vi "Lighthouse Monitoring & Control System 3.vi"() -> ()   [LabVIEW 2012]
uses:
  <vilib>/DAQmx/read.llb/DAQmx Read (Counter DBL 1Chan 1Samp).vi
  <vilib>/DAQmx/write.llb/DAQmx Write (Digital U8 1Chan 1Samp).vi
  <vilib>/DAQmx/write.llb/DAQmx Write (Digital 1D Bool NChan 1Samp 1Line).vi
  <vilib>/DAQmx/write.llb/DAQmx Write (Analog DBL 1Chan 1Samp).vi
  <vilib>/DAQmx/read.llb/DAQmx Read (Analog DBL 1Chan 1Samp).vi
  <vilib>/DAQmx/create/channels.llb/DAQmx Create Channel (CI-Count Edges).vi
  <vilib>/DAQmx/create/channels.llb/DAQmx Create Channel (DO-Digital Output).vi
  <vilib>/DAQmx/create/channels.llb/DAQmx Create Channel (AI-Voltage-Basic).vi
  <vilib>/DAQmx/create/channels.llb/DAQmx Create Channel (AO-Voltage-Basic).vi
  <vilib>/DAQmx/miscellaneous.llb/DAQmx Fill In Error Info.vi
panel:
  out "Array":bool[](array[boolean])
  out "Data to Write":u32=255 format="%x"
  out "Voltage":dbl
  in  "?":bool
  out "Slot Count":dbl
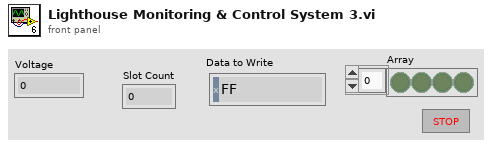
[diagram p1: front panel]
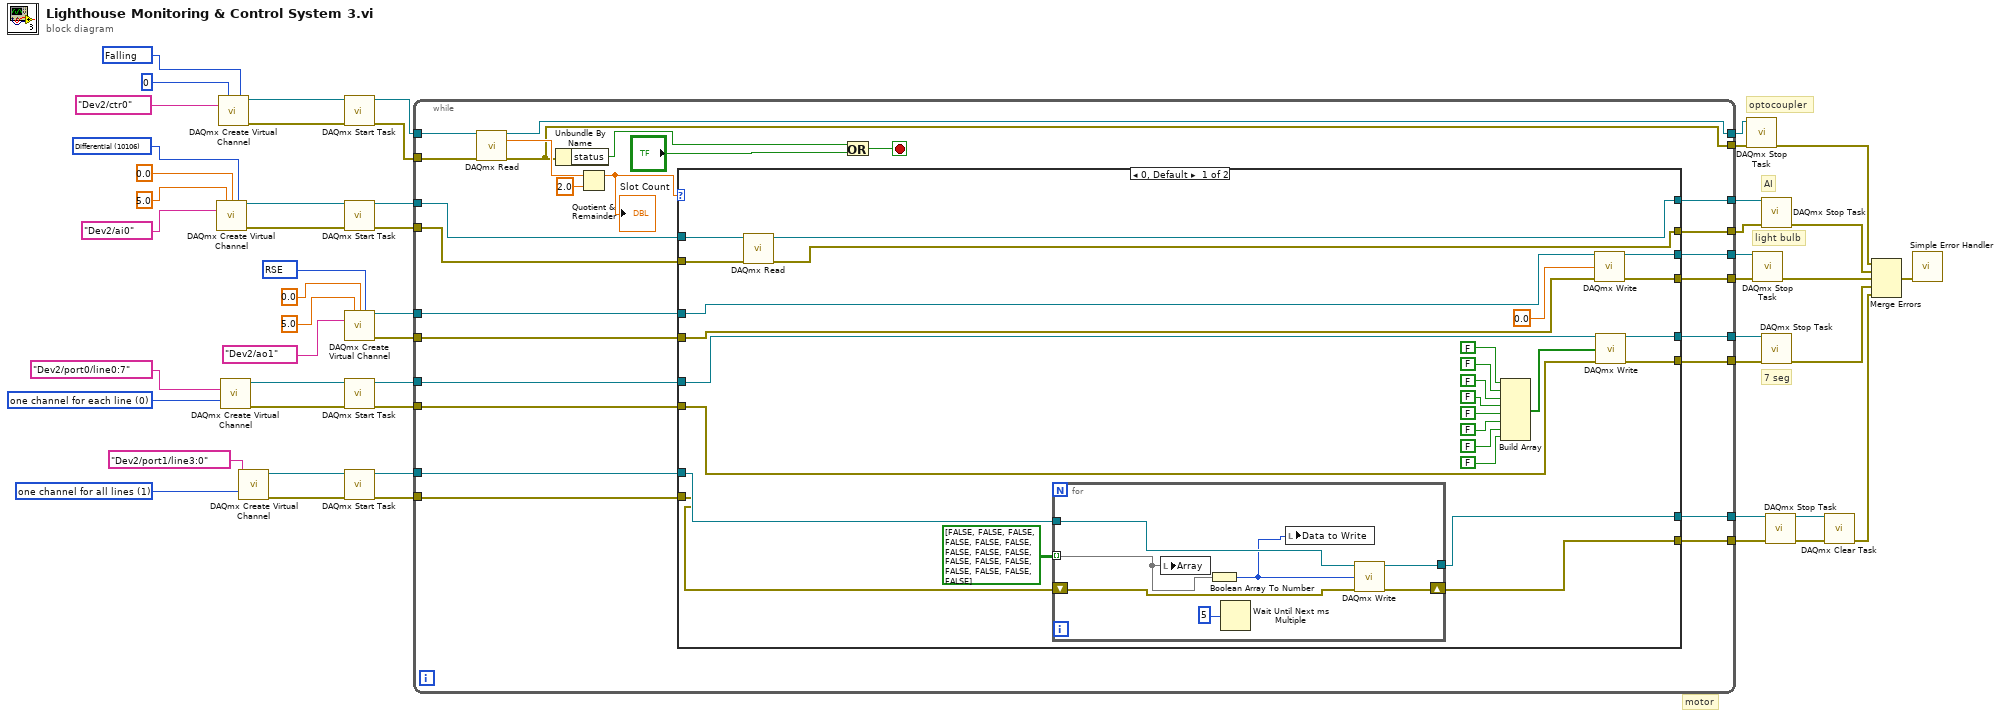
[diagram p0: block diagram]
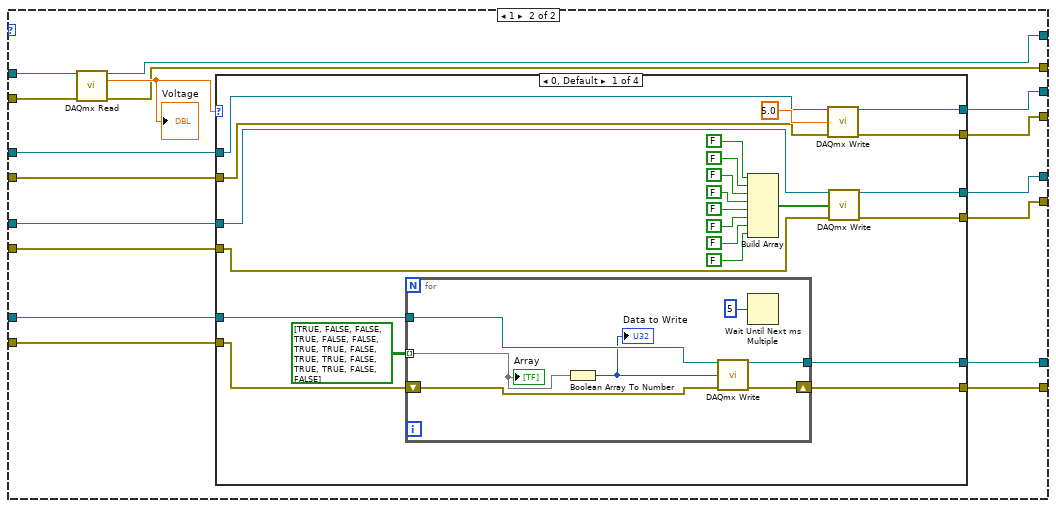
[diagram p2: hidden frame]
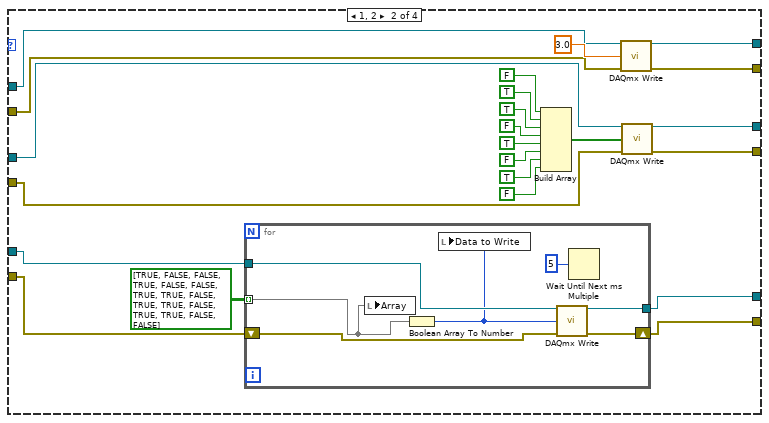
[diagram p3: hidden frame]
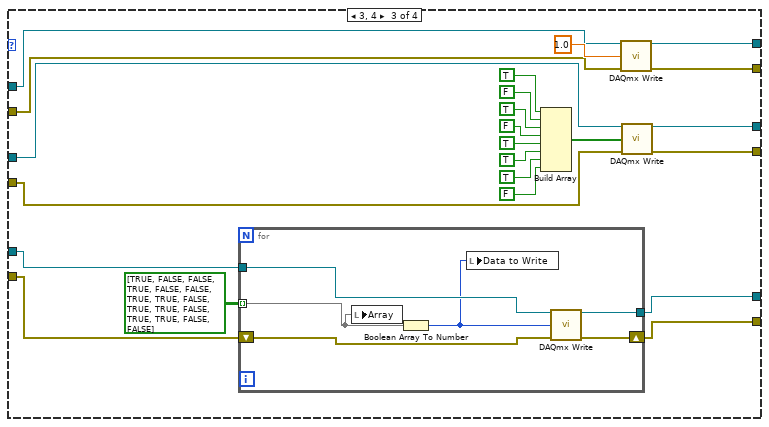
[diagram p4: hidden frame]
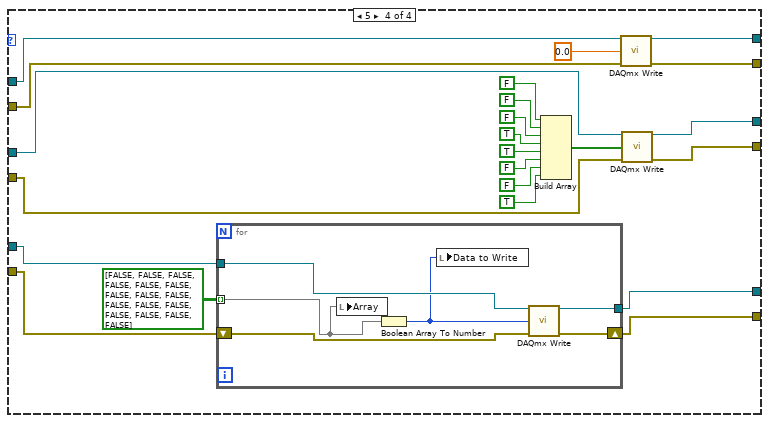
[diagram p5: hidden frame]
diagram:
  w11 = 1 items=["one channel for each line", "one channel for all lines"] ("line grouping")
  w38 = 0 items=["one channel for each line", "one channel for all lines"] ("line grouping")
  w41 = 10083 items=["Default"=-1, "RSE"=10083, "Differential"=10106, "Pseudodifferential"=12529] ("output terminal configuration")
  w44 = 10106 items=["default"=-1, "RSE"=10083, "NRSE"=10078, "Differential"=10106, "Pseudodifferential"=12529] ("input terminal configuration")
  w51 = 10171 items=["Rising"=10280, "Falling"=10171] ("edge")
  # "motor"
  # "7 seg"
  # "AI"
  # "light bulb"
  # "optocoupler"
  n1 = call-poly <vilib>:"DAQmx Create Virtual Channel.vi"("maximum value"=5.0, "minimum value"=0.0, "input terminal configuration"=w44, "physical channels"=tag "Dev2/ai0") -> ("task out"=w42:refnum<k21>, "error out"=w43:errorcluster)  [unwired: 10 in]
  n2 = call-poly <vilib>:"DAQmx Create Virtual Channel.vi"("initial count"=u32 0, "edge"=w51, "counter"=tag "Dev2/ctr0") -> ("task out"=w50:refnum<k21>, "error out"=w49:errorcluster)  [unwired: 11 in]
  n3 = call-poly <vilib>:"DAQmx Create Virtual Channel.vi"("lines"=tag "Dev2/port0/line0:7", "line grouping"=w38) -> ("task out"=w37:refnum<k21>, "error out"=w36:errorcluster)  [unwired: 12 in]
  n4 = call-poly <vilib>:"DAQmx Create Virtual Channel.vi"("lines"=tag "Dev2/port1/line3:0", "line grouping"=w11) -> ("task out"=w10:refnum<k21>, "error out"=w9:errorcluster)  [unwired: 12 in]
  n5 = call <vilib>:"DAQmx Start Task.vi"("task/channels in"=w50, "error in"=w49) -> ("task out"=w46:refnum<k21>, "error out"=w45:errorcluster)  [unwired: 12 in]
  n6 = call <vilib>:"DAQmx Start Task.vi"("task/channels in"=w42, "error in"=w43) -> ("task out"=w32:refnum<k21>, "error out"=w31:errorcluster)  [unwired: 12 in]
  n7 = call-poly <vilib>:"DAQmx Create Virtual Channel.vi"("maximum value"=5.0, "minimum value"=0.0, "output terminal configuration"=w41, "physical channels"=tag "Dev2/ao1") -> ("task out"=w30:refnum<k21>, "error out"=w29:errorcluster)  [unwired: 10 in]
  n8 = call <vilib>:"DAQmx Start Task.vi"("task/channels in"=w37, "error in"=w36) -> ("task out"=w28:refnum<k21>, "error out"=w27:errorcluster)  [unwired: 12 in]
  n9 = call <vilib>:"DAQmx Start Task.vi"("task/channels in"=w10, "error in"=w9) -> ("task out"=w8:refnum<k21>, "error out"=w7:errorcluster)  [unwired: 12 in]
  n10 = while {
    tunnel: w46 -> [w77]
    tunnel: w45 -> [w76]
    tunnel: [w64] -> w34
    tunnel: w32 -> [w70]
    tunnel: w31 -> [w69]
    tunnel: w30 -> [w68]
    tunnel: w29 -> [w67]
    tunnel: w28 -> [w66]
    tunnel: w27 -> [w65]
    tunnel: [w63] -> w22
    tunnel: [w62] -> w21
    tunnel: [w61] -> w20
    tunnel: [w60] -> w19
    tunnel: [w59] -> w18
    tunnel: [w58] -> w17
    tunnel: [w57] -> w16
    tunnel: w8 -> [w55]
    tunnel: w7 -> [w54]
    tunnel: [w52] -> w3
    tunnel: [w53] -> w2
    stop <- w73 stop-if-true
    n11 = call-poly <vilib>:"DAQmx Read.vi"("task/channels in"=w77, "error in"=w76) -> ("task out"=w64:refnum<k21>, "data"=w75:dbl, "error out"=w63:errorcluster)  [unwired: 11 in]
    n12 = Unbundle By Name(w63) -> ("status"=w72:bool)
    n13 = Quotient & Remainder(x=w75, y=2.0) -> (x-y*floor(x/y)=w56:dbl)  [unwired: 1 out]
    "Slot Count" <- w56
    n14 = case shown="0, Default" w56 {
      tunnel: w70 -> [w101 w127]
      tunnel: w69 -> [w100 w126]
      tunnel: w68 -> [w99 w125]
      tunnel: w67 -> [w98 w124]
      tunnel: w66 -> [w103 w123]
      tunnel: w65 -> [w102 w122]
      tunnel: [w95 w121] -> w58
      tunnel: [w96 w120] -> w62
      tunnel: [w97 w119] -> w61
      tunnel: [w92 w118] -> w60
      tunnel: [w93 w117] -> w59
      tunnel: [w94 w116] -> w57
      tunnel: w55 -> [w81 w115]
      tunnel: w54 -> [w80 w114]
      tunnel: [w78 w112] -> w53
      tunnel: [w79 w113] -> w52
      frame 0, Default {
        n15 = call-poly <vilib>:"DAQmx Read.vi"("task/channels in"=w101, "error in"=w100) -> ("task out"=w94:refnum<k21>, "error out"=w97:errorcluster)  [unwired: 11 in, 1 out]
        n16 = for {
          tunnel: w81 -> [w110]
          tunnel: [w109] -> w79
          shift-right: [w107] -> w78
          shift-left: w80 -> [w111]
          tunnel: bool[][] [[FALSE, FALSE, FALSE, FALSE], [FALSE, FALSE, FALSE, FALSE], [FALSE, FALSE, FALSE, FALSE], [FALSE, FALSE, FALSE, FALSE]] -> [w105] mode=indexing
          n17 = local write "Array"(w105) -> ()
          n18 = Boolean Array To Number(Boolean array=w105) -> (number=w106:u32)
          n19 = Wait Until Next ms Multiple(millisecond multiple=5) -> ()  [unwired: 1 out]
          n20 = local write "Data to Write"(w106) -> ()
          n21 = call-poly <vilib>:"DAQmx Write.vi"("task/channels in"=w110, "data"=w106, "error in"=w111) -> ("task out"=w109:refnum<k21>, "error out"=w107:errorcluster)  [unwired: 10 in, 1 out]
        }
        n22 = Build Array(FALSE, FALSE, FALSE, FALSE, FALSE, FALSE, FALSE, FALSE) -> (w83:bool[])
        n23 = call-poly <vilib>:"DAQmx Write.vi"("task/channels in"=w99, "data"=0.0, "error in"=w98) -> ("task out"=w95:refnum<k21>, "error out"=w96:errorcluster)  [unwired: 10 in, 1 out]
        n24 = call-poly <vilib>:"DAQmx Write.vi"("task/channels in"=w103, "data"=w83, "error in"=w102) -> ("task out"=w93:refnum<k21>, "error out"=w92:errorcluster)  [unwired: 10 in, 1 out]
      }
      frame 1 {
        n25 = call-poly <vilib>:"DAQmx Read.vi"("task/channels in"=w127, "error in"=w126) -> ("task out"=w116:refnum<k21>, "data"=w128:dbl, "error out"=w119:errorcluster)  [unwired: 11 in]
        "Voltage" <- w128
        n26 = case shown="0, Default" w128 {
          tunnel: w125 -> [w137 w171 w201 w230]
          tunnel: w124 -> [w136 w170 w200 w229]
          tunnel: [w141 w169 w199 w228] -> w121
          tunnel: [w140 w168 w198 w227] -> w120
          tunnel: [w139 w167 w197 w226] -> w117
          tunnel: [w138 w166 w196 w225] -> w118
          tunnel: w123 -> [w135 w165 w195 w224]
          tunnel: w122 -> [w134 w164 w194 w223]
          tunnel: w115 -> [w133 w162 w192 w221]
          tunnel: w114 -> [w132 w161 w191 w220]
          tunnel: [w131 w160 w190 w219] -> w113
          tunnel: [w130 w159 w189 w218] -> w112
          frame 0, Default {
            n27 = for {
              tunnel: w133 -> [w157]
              tunnel: [w156] -> w131
              shift-right: [w155] -> w130
              shift-left: w132 -> [w158]
              tunnel: bool[][] [[TRUE, FALSE, FALSE, TRUE], [FALSE, FALSE, TRUE, TRUE], [FALSE, TRUE, TRUE, FALSE], [TRUE, TRUE, FALSE, FALSE]] -> [w153] mode=indexing
              n28 = Boolean Array To Number(Boolean array=w153) -> (number=w154:u32)
              "Data to Write" <- w154
              n29 = call-poly <vilib>:"DAQmx Write.vi"("task/channels in"=w157, "data"=w154, "error in"=w158) -> ("task out"=w156:refnum<k21>, "error out"=w155:errorcluster)  [unwired: 10 in, 1 out]
              n30 = Wait Until Next ms Multiple(millisecond multiple=u32 5) -> ()  [unwired: 1 out]
              "Array" <- w153
            }
            n31 = Build Array(FALSE, FALSE, FALSE, FALSE, FALSE, FALSE, FALSE, FALSE) -> (w142:bool[])
            n32 = call-poly <vilib>:"DAQmx Write.vi"("task/channels in"=w137, "data"=5.0, "error in"=w136) -> ("task out"=w141:refnum<k21>, "error out"=w140:errorcluster)  [unwired: 10 in, 1 out]
            n33 = call-poly <vilib>:"DAQmx Write.vi"("task/channels in"=w135, "data"=w142, "error in"=w134) -> ("task out"=w139:refnum<k21>, "error out"=w138:errorcluster)  [unwired: 10 in, 1 out]
          }
          frame 1, 2 {
            n34 = for {
              tunnel: w162 -> [w183]
              tunnel: [w187] -> w160
              shift-right: [w186] -> w159
              shift-left: w161 -> [w188]
              tunnel: bool[][] [[TRUE, FALSE, FALSE, TRUE], [FALSE, FALSE, TRUE, TRUE], [FALSE, TRUE, TRUE, FALSE], [TRUE, TRUE, FALSE, FALSE]] -> [w184] mode=indexing
              n35 = local write "Array"(w184) -> ()
              n36 = Boolean Array To Number(Boolean array=w184) -> (number=w182:u32)
              n37 = local write "Data to Write"(w182) -> ()
              n38 = call-poly <vilib>:"DAQmx Write.vi"("task/channels in"=w183, "data"=w182, "error in"=w188) -> ("task out"=w187:refnum<k21>, "error out"=w186:errorcluster)  [unwired: 10 in, 1 out]
              n39 = Wait Until Next ms Multiple(millisecond multiple=u32 5) -> ()  [unwired: 1 out]
            }
            n40 = Build Array(FALSE, TRUE, TRUE, FALSE, TRUE, FALSE, TRUE, FALSE) -> (w172:bool[])
            n41 = call-poly <vilib>:"DAQmx Write.vi"("task/channels in"=w171, "data"=3.0, "error in"=w170) -> ("task out"=w169:refnum<k21>, "error out"=w168:errorcluster)  [unwired: 10 in, 1 out]
            n42 = call-poly <vilib>:"DAQmx Write.vi"("task/channels in"=w165, "data"=w172, "error in"=w164) -> ("task out"=w167:refnum<k21>, "error out"=w166:errorcluster)  [unwired: 10 in, 1 out]
          }
          frame 3, 4 {
            n43 = for {
              tunnel: w192 -> [w216]
              tunnel: [w215] -> w190
              shift-right: [w214] -> w189
              shift-left: w191 -> [w217]
              tunnel: bool[][] [[TRUE, FALSE, FALSE, TRUE], [FALSE, FALSE, TRUE, TRUE], [FALSE, TRUE, TRUE, FALSE], [TRUE, TRUE, FALSE, FALSE]] -> [w213] mode=indexing
              n44 = local write "Array"(w213) -> ()
              n45 = Boolean Array To Number(Boolean array=w213) -> (number=w212:u32)
              n46 = local write "Data to Write"(w212) -> ()
              n47 = call-poly <vilib>:"DAQmx Write.vi"("task/channels in"=w216, "data"=w212, "error in"=w217) -> ("task out"=w215:refnum<k21>, "error out"=w214:errorcluster)  [unwired: 10 in, 1 out]
            }
            n48 = Build Array(TRUE, FALSE, TRUE, FALSE, TRUE, TRUE, TRUE, FALSE) -> (w202:bool[])
            n49 = call-poly <vilib>:"DAQmx Write.vi"("task/channels in"=w201, "data"=1.0, "error in"=w200) -> ("task out"=w199:refnum<k21>, "error out"=w198:errorcluster)  [unwired: 10 in, 1 out]
            n50 = call-poly <vilib>:"DAQmx Write.vi"("task/channels in"=w195, "data"=w202, "error in"=w194) -> ("task out"=w197:refnum<k21>, "error out"=w196:errorcluster)  [unwired: 10 in, 1 out]
          }
          frame 5 {
            n51 = for {
              tunnel: w221 -> [w245]
              tunnel: [w244] -> w219
              shift-right: [w243] -> w218
              shift-left: w220 -> [w246]
              tunnel: bool[][] [[FALSE, FALSE, FALSE, FALSE], [FALSE, FALSE, FALSE, FALSE], [FALSE, FALSE, FALSE, FALSE], [FALSE, FALSE, FALSE, FALSE]] -> [w242] mode=indexing
              n52 = local write "Array"(w242) -> ()
              n53 = Boolean Array To Number(Boolean array=w242) -> (number=w241:u32)
              n54 = local write "Data to Write"(w241) -> ()
              n55 = call-poly <vilib>:"DAQmx Write.vi"("task/channels in"=w245, "data"=w241, "error in"=w246) -> ("task out"=w244:refnum<k21>, "error out"=w243:errorcluster)  [unwired: 10 in, 1 out]
            }
            n56 = Build Array(FALSE, FALSE, FALSE, TRUE, TRUE, FALSE, FALSE, TRUE) -> (w231:bool[])
            n57 = call-poly <vilib>:"DAQmx Write.vi"("task/channels in"=w230, "data"=0.0, "error in"=w229) -> ("task out"=w228:refnum<k21>, "error out"=w227:errorcluster)  [unwired: 10 in, 1 out]
            n58 = call-poly <vilib>:"DAQmx Write.vi"("task/channels in"=w224, "data"=w231, "error in"=w223) -> ("task out"=w226:refnum<k21>, "error out"=w225:errorcluster)  [unwired: 10 in, 1 out]
          }
        }
      }
    }
    n59 = Or(x=w72, y="?") -> (x .or. y?=w73:bool)
  }
  n60 = call <vilib>:"DAQmx Stop Task.vi"("task/channels in"=w34, "error in"=w22) -> ("error out"=w33:errorcluster)  [unwired: 12 in, 1 out]
  n61 = call <vilib>:"DAQmx Stop Task.vi"("task/channels in"=w17, "error in"=w21) -> ("error out"=w25:errorcluster)  [unwired: 12 in, 1 out]
  n62 = call <vilib>:"DAQmx Stop Task.vi"("task/channels in"=w16, "error in"=w20) -> ("error out"=w26:errorcluster)  [unwired: 12 in, 1 out]
  n63 = call <vilib>:"DAQmx Stop Task.vi"("task/channels in"=w18, "error in"=w19) -> ("error out"=w24:errorcluster)  [unwired: 12 in, 1 out]
  n64 = call <vilib>:"DAQmx Stop Task.vi"("task/channels in"=w3, "error in"=w2) -> ("task out"=w6:refnum<k21>, "error out"=w5:errorcluster)  [unwired: 12 in]
  n65 = call <vilib>:"DAQmx Clear Task.vi"("task in"=w6, "error in"=w5) -> ("error out"=w4:errorcluster)  [unwired: 13 in]
  n66 = Merge Errors(w33, w26, w25, w24, w4) -> (w23:errorcluster)
  n67 = call <vilib>:"Simple Error Handler.vi"("error in (no error)"=w23) -> ()  [unwired: 4 in, 5 out]
